vi "Set Transaction.vi"(8 "error in (no error)":errorcluster, 10 "Transactions":T1, 11 "ATM Controller in":refnum<class "ATM Controller.lvclass">) -> (0 "error out":errorcluster, 3 "ATM Controller out":refnum<class "ATM Controller.lvclass">)   [LabVIEW 2019, in "ATM Controller.lvlib" / "ATM Controller.lvclass"]
uses:
  ATM Controller.lvclass
  Sim User Console Actor/ATM Controller/Transactions -Cluster.ctl
  ATM Controller.lvclass/ATM Controller.ctl
  Sim Display Console Actor/Sim Display Console Actor Messages/Write Transaction Msg/Write Transaction Msg.lvclass/Write Transaction Msg.ctl
  <vilib>/ActorFramework/Message Enqueuer/Message Enqueuer.lvclass/Message Enqueuer.ctl
  <vilib>/ActorFramework/Message Enqueuer/Enqueue.vi
  Sim Display Console Actor/Sim Display Console Actor Messages/Write Transaction Msg/Write Transaction Msg.lvclass
  C:/Program Files (x86)/National Instruments/LabVIEW 2019/vi.lib/ActorFramework/Message/Message.lvclass
  <vilib>/ActorFramework/Message Priority Queue/Priority Enqueue.vi
  Sim User Console Actor/ATM Controller/Sim User Console Actor.lvclass
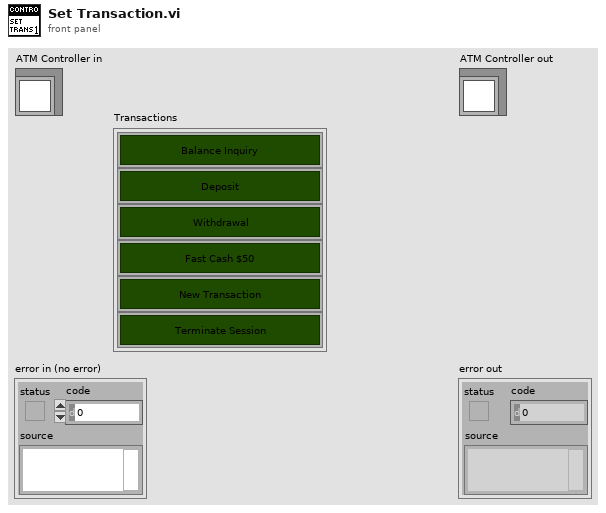
[diagram p1: front panel]
types:
  T1 = typedef "Sim User Console Actor.lvlib/Sim User Console Actor.lvclass/Transactions -Cluster.ctl" = cluster{"Balance Inquiry":bool, "Deposit":bool, "Withdrawal":bool, "Fast Cash $50":bool, "New Transaction":bool, "Terminate Session":bool}
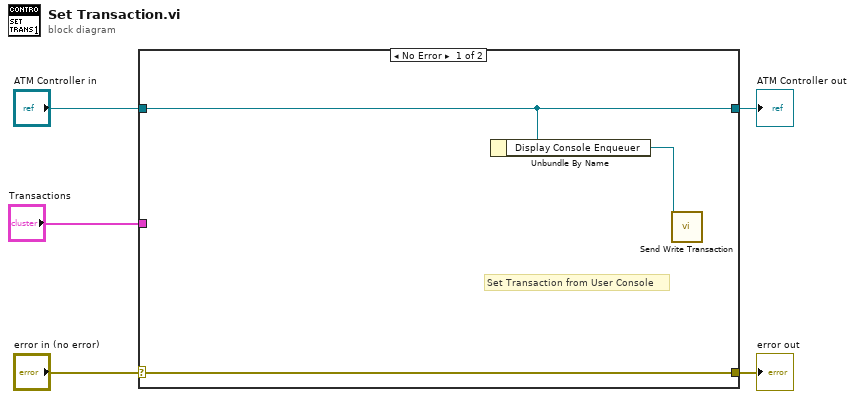
[diagram p0: block diagram]
diagram:
  n1 = case shown="No Error" "error in (no error)" {
    selector: "error in (no error)" -> [w8 w10]
    tunnel: [w8 w10] -> w4
    tunnel: [w7 w9] -> w2
    tunnel: "ATM Controller in" -> [w7 w9]
    tunnel: "Transactions" -> [_ _]
    frame No Error {
      # "Set Transaction from User Console"
      n2 = Unbundle By Name(w7) -> ("Display Console Enqueuer"=w6:refnum<class "Message Enqueuer.lvclass">)
      n3 = call "Send Write Transaction.vi"("Message Enqueuer"=w6) -> ()  [unwired: 9 in, 2 out]
    }
    frame Error {
    }
  }
  "error out" <- w4
  "ATM Controller out" <- w2
